vi "get_call_chain.vi"(3 "Remove lvlib names (F)":bool, 5 "Cut first x elements\nfrom Error Chain (0)":i32) -> (0 "ExVI index":i32, 1 "Call chain out in spreadsheet string":string, 2 "Call chain out":string[](array[string]))   [LabVIEW 2014, in "rszvl_rsidr_core.lvlib"]
uses:
  rszvl_rsidr_core.lvlib
  Match Regular Expression.xnode
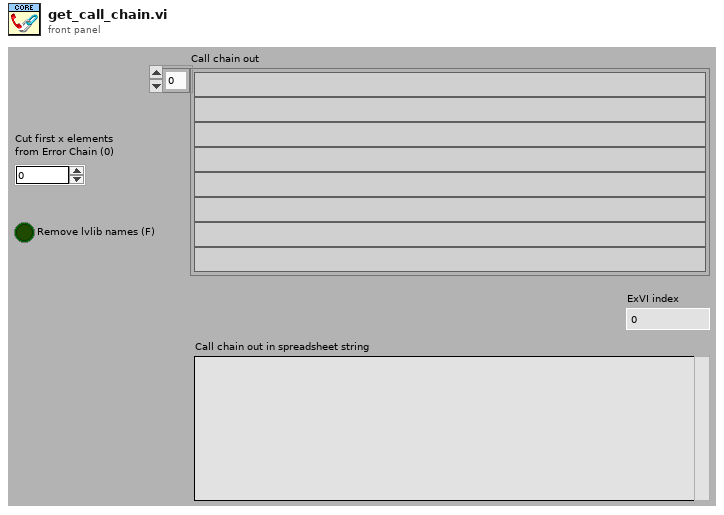
[diagram p1: front panel]
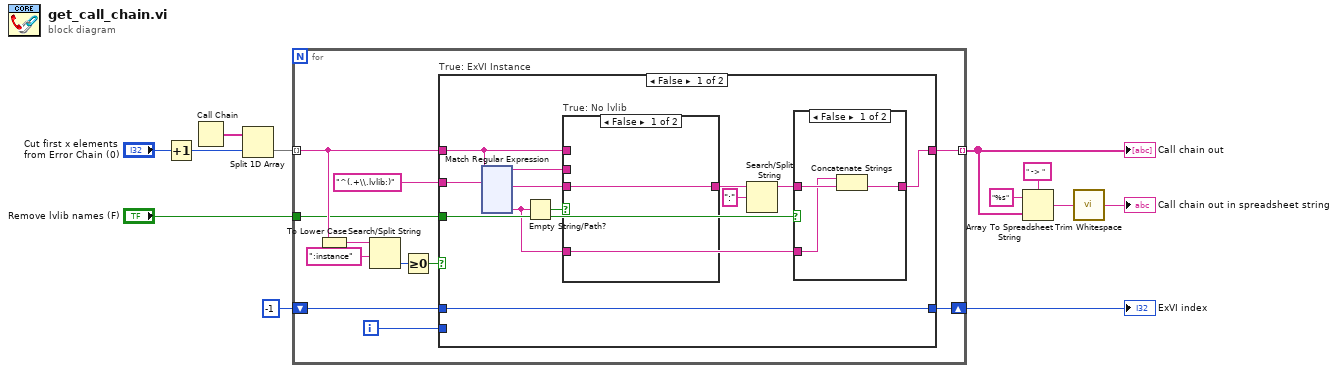
[diagram p0: block diagram]
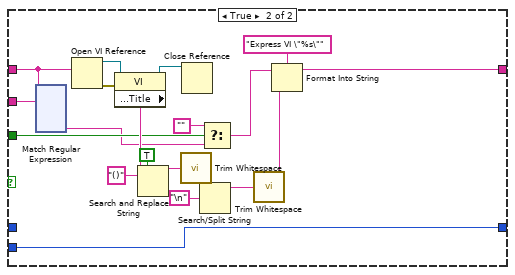
[diagram p4: hidden frame]
diagram:
  n1 = Increment(x="Cut first x elements\nfrom Error Chain (0)") -> (x+1=w7:i32)
  n2 = Call Chain() -> (call chain=w11:string[])
  n3 = Split 1D Array(array=w11, index=w7) -> (second subarray=w10:string[])  [unwired: 1 out]
  n4 = for {
    tunnel: w10 -> [w19] mode=indexing
    tunnel: [w18] -> w6 mode=indexing
    shift-right: [w14] -> w8
    shift-left: -1 -> [w16]
    tunnel: "Remove lvlib names (F)" -> [w13]
    i -> [w15]
    n5 = To Lower Case(string=w19) -> (all lower case string=w20:string)
    n6 = Search/Split String(string=w20, search string/char (-)=":instance") -> (offset of match=w22:i32)  [unwired: 1 in, 2 out]
    n7 = Greater Or Equal To 0?(x=w22) -> (x >= 0?=w17:bool)
    n8 = case "True: ExVI Instance" shown="False" w17 {
      tunnel: w19 -> [w33 w162]
      tunnel: "^(.+\\.lvlib:)" ("search string/char (-)") -> [w34 w161]
      tunnel: [w25 w160] -> w18
      tunnel: w16 -> [w35 _]
      tunnel: w15 -> [_ w159]
      tunnel: [w35 w159] -> w14
      tunnel: w13 -> [w27 w158]
      frame False {
        n9 = xnode ("Match Regular Expression")("input string"=w33, "regular expression"=w34) -> ("before match"=w30:string, "after match"=w31:string, "submatch 1"=w24:string)  [unwired: 4 in, 3 out]
        n10 = Empty String/Path?(string/path=w24) -> (empty?=w32:bool)
        n11 = case "True: No lvlib" shown="False" w32 {
          tunnel: w33 -> [_ w41]
          tunnel: w31 -> [w40 _]
          tunnel: [w40 w41] -> w28
          tunnel: w30 -> [_ _]
          tunnel: w24 -> [_ _]
          frame False {
          }
          frame True {
          }
        }
        n12 = Search/Split String(string=w28, search string/char (-)=":") -> (substring before match=w26:string)  [unwired: 1 in, 2 out]
        n13 = case shown="False" w27 {
          tunnel: w26 -> [w38 w39]
          tunnel: [w37 w39] -> w25
          tunnel: w24 -> [w36 _]
          frame False {
            n14 = Concatenate Strings(w36, w38) -> (w37:string)
          }
          frame True {
          }
        }
      }
      frame True {
        n15 = xnode ("Match Regular Expression")("input string"=w162, "regular expression"=w161) -> ("submatch 1"=w157:string)  [unwired: 4 in, 5 out]
        n16 = Open VI Reference(vi path=w162) -> (vi reference=w164:refnum<vi>, error out=w173:errorcluster)  [unwired: 5 in]
        n17 = property on="Property Node" class="VI"(reference=w164, error in=w173) -> (reference out=w174:refnum<vi>, "Front Panel Window:Title"=w167:string)  [unwired: 1 out]
        n18 = Search and Replace String(replace all?=TRUE ("replace all? (F)"), input string=w167, search string="()") -> (result string=w170:string)  [unwired: 5 in, 3 out]
        n19 = call "Trim Whitespace.vi"("string"=w170) -> ("trimmed string"=w171:string)  [unwired: 1 in]
        n20 = Close Reference(reference=w174) -> ()  [unwired: 1 in, 1 out]
        n21 = Search/Split String(string=w171, search string/char (-)="\n" ("Line Feed Constant")) -> (substring before match=w166:string)  [unwired: 1 in, 2 out]
        n22 = Select(t="" ("Empty String Constant"), s=w158, f=w157) -> (s? t:f=w156:string)
        n23 = call "Trim Whitespace.vi"("string"=w166) -> ("trimmed string"=w163:string)  [unwired: 1 in]
        n24 = Format Into String(format string="Express VI \"%s\"", initial string=w156, w163) -> (resulting string=w160:string)  [unwired: 1 in, 1 out]
      }
    }
  }
  "Call chain out" <- w6
  "ExVI index" <- w8
  n25 = Array To Spreadsheet String(delimiter (Tab)=" -> ", array=w6, 3:"%s" ("format string")) -> (spreadsheet string=w3:string)
  n26 = call "Trim Whitespace.vi"("string"=w3) -> ("trimmed string"=→"Call chain out in spreadsheet string":string)  [unwired: 1 in]
